vi "Get Y.vi"(8 "error in (no error)":errorcluster, 11 "SR7270 Drivers in":refnum<class "SR7270 Drivers.lvclass">) -> (0 "error out":errorcluster, 2 "Y (V or A)":dbl, 3 "SR7270 Drivers out":refnum<class "SR7270 Drivers.lvclass">)   [LabVIEW 2016, in "SR7270 Drivers.lvclass"]
uses:
  SR7270 Drivers.lvclass
  SR7270 Drivers.lvclass/SR7270 Drivers.ctl
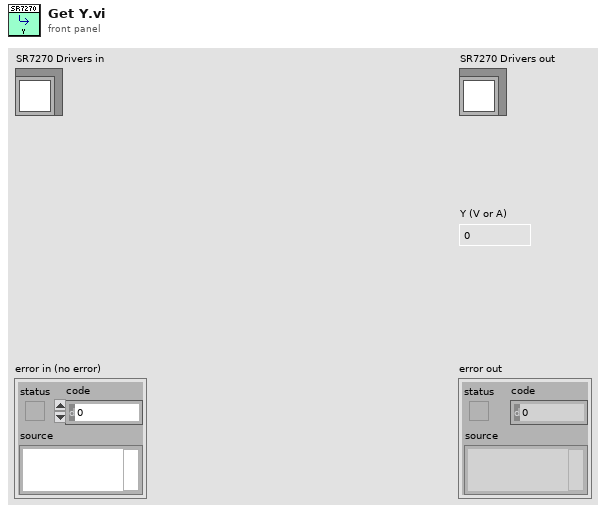
[diagram p1: front panel]
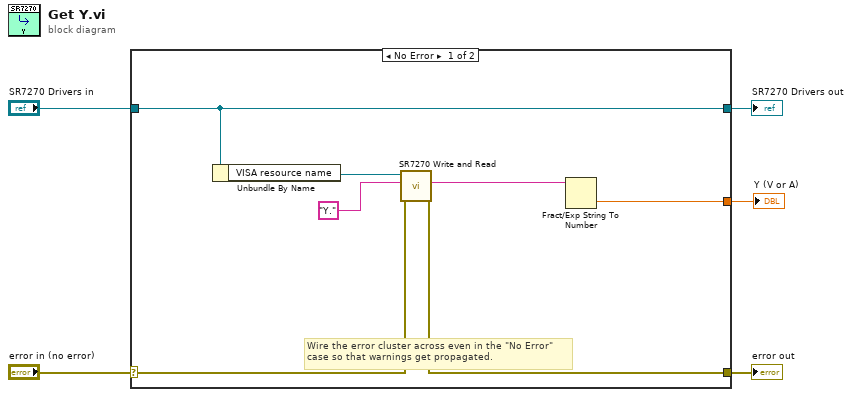
[diagram p0: block diagram]
diagram:
  n1 = case shown="No Error" "error in (no error)" {
    selector: "error in (no error)" -> [w10 w14]
    tunnel: [w9 w14] -> w4
    tunnel: [w11 w13] -> w2
    tunnel: "SR7270 Drivers in" -> [w11 w13]
    tunnel: [w6 _] -> w1
    frame No Error {
      # "Wire the error cluster across even in the \"No Error\"\ncase so that warnings get propagated."
      n2 = Unbundle By Name(w11) -> ("VISA resource name"=w12:refnum<visa-resource-name>)
      n3 = call "SR7270 Write and Read.vi"("error in (no error)"=w10, "Command Name"="Y.", "VISA resource name"=w12) -> ("error out"=w9:errorcluster, "Read"=w7:string)  [unwired: 5 in, 2 out]
      n4 = Fract/Exp String To Number(string=w7) -> (number=w6:dbl)  [unwired: 3 in, 1 out]
    }
    frame Error {
    }
  }
  "error out" <- w4
  "SR7270 Drivers out" <- w2
  "Y (V or A)" <- w1
